vi "CVI_TD_PopUp Menu_Items.vi"() -> (0 "Array":T1[](array[typedef]) {"uFlags" items=["MF_STRING"=0, "MF_GRAYED"=1, "MF_DISABLED"=2, "MF_CHECKED"=8, "MF_HILITE"=128, "MF_POPUP"=16, "MF_SEPARATOR"=2048]}, 1 "?":T1 {"uFlags" items=["MF_STRING"=0, "MF_GRAYED"=1, "MF_DISABLED"=2, "MF_CHECKED"=8, "MF_HILITE"=128, "MF_POPUP"=16, "MF_SEPARATOR"=2048]})   [LabVIEW 2013]
uses:
  TD_PopUp Menu_Items.ctl
  TD_PopUp Menu_Flags.ctl
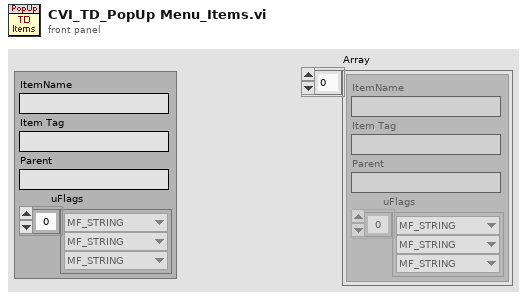
[diagram p1: front panel]
types:
  T1 = typedef "TD_PopUp Menu_Items.ctl" = cluster{"ItemName":string, "Item Tag":string, "Parent":string, "uFlags":T2[]}
  T2 = typedef "TD_PopUp Menu_Flags.ctl" = u32
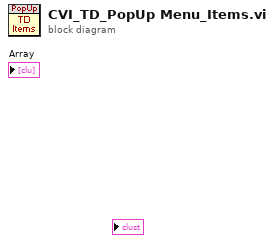
[diagram p0: block diagram]
diagram:
